vi "DAQConfig.vi"() -> ()   [LabVIEW 2017, in "DAQConfig.lvlib"]
uses:
  DAQConfig.lvlib
  Communication/SubVIs/QueueRepo.Action.ctl
  Main/GUIReferences.Action.ctl
  <vilib>/Utility/miscctls.llb/LVPointTypeDef.ctl
  Communication/Communication.lvlib
  Main/MainGUI.lvlib
panel:
  in  "Start Button":bool
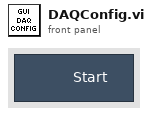
[diagram p1: front panel]
types:
  T1 = typedef "Communication.lvlib/QueueRepo.Action.ctl" = enum16{"Add", "Get", "Destroy", "Get All", "Clear"}
  T2 = typedef "LVPointTypeDef.ctl" = cluster{"Horizontal":i16, "Vertical":i16}
  T3 = typedef "MainGUI.lvlib/GUIReferences.Action.ctl" = enum16{"Get", "Register", "Unregister"}
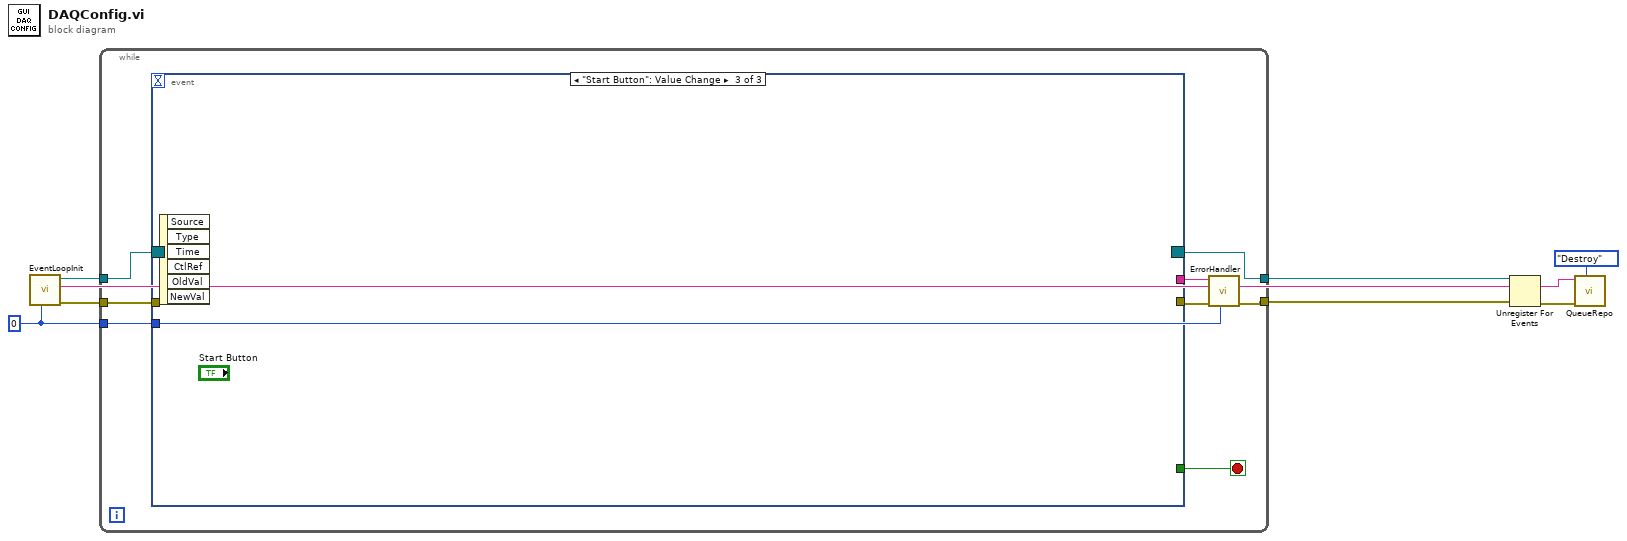
[diagram p0: block diagram]
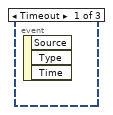
[diagram p2: hidden frame]
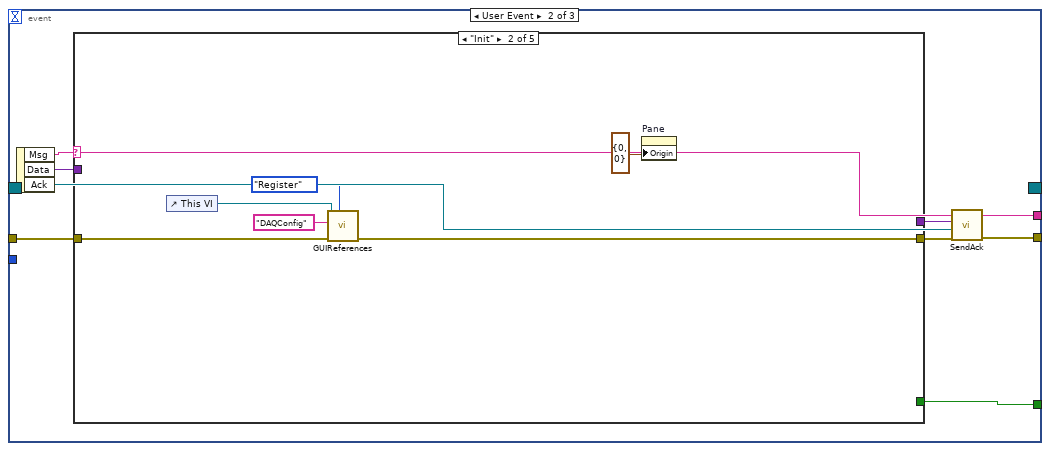
[diagram p3: hidden frame]
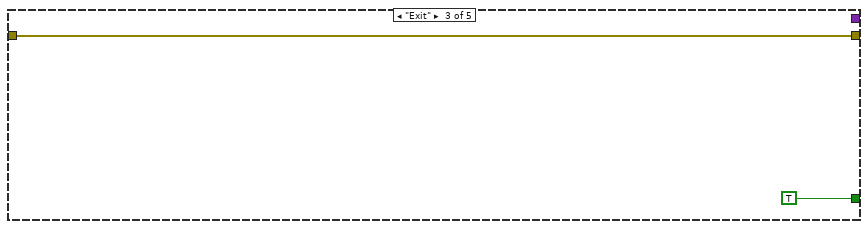
[diagram p5: hidden frame]
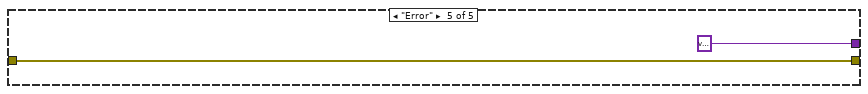
[diagram p7: hidden frame]
diagram:
  w6 = 0 ("Instance")
  n1 = call "EventLoopInit.vi"("Instance"=w6) -> ("error out"=w7:errorcluster, "Loop Name"=w3:string, "Event Registration Refnum"=w8:refnum<event-registration>)  [unwired: 8 in]
  n2 = while {
    tunnel: w8 -> [w16]
    tunnel: w7 -> [w15]
    tunnel: w6 -> [w10]
    tunnel: [w13] -> w5
    tunnel: [w12] -> w4
    stop <- w14 stop-if-true
    n3 = event shown="[2] \"Start Button\": Value Change" {
      selector: w16 -> [_ _ _]
      dyn-events: [_ _ _] -> w13
      timeout: _ -> [_ _ _]
      tunnel: w15 -> [_ w23 _]
      tunnel: [_ w17 _] -> w11
      tunnel: w10 -> [_ _ _]
      tunnel: [_ w19 _] -> w14
      tunnel: [_ w18 _] -> w9
      event Timeout {
        n4 = event-data() -> ()  [unwired: 1 in, 3 out]
      }
      event User Event {
        n5 = event-data() -> ("Msg"=w18:string, "Data"=w24:variant, "Ack"=w22:refnum<notifier>)  [unwired: 1 in]
        n6 = case shown="\"Init\"" w18 {
          tunnel: w24 -> [_ _ _ _ _]
          tunnel: w23 -> [w25 w31 w33 w34 w35]
          tunnel: [_ _ _ _ variant] -> w21
          tunnel: [w25 w30 w33 w34 w35] -> w20
          tunnel: [_ _ TRUE _ _] -> w19
          frame Default {
          }
          frame "Init" {
            n7 = control-ref of="This VI"() -> (w28:refnum<vi>)
            n8 = call "GUIReferences.vi"("Action"=GUIReferences.Action."Register", "error in (no error)"=w31, "String"="DAQConfig", "VI Refnum"=w28) -> ("error out"=w30:errorcluster)  [unwired: 6 in, 1 out]
            n9 = property on="Pane" class="Pane"("Origin"=T2 {"Horizontal"=0, "Vertical"=0}) -> ()  [unwired: 2 in, 2 out]
          }
          frame "Exit" {
          }
          frame "Tick" {
          }
          frame "Error" {
          }
        }
        n10 = call "SendAck.vi"("error in (no error)"=w20, "Ack"=w22, "Variant"=w21) -> ("error out"=w17:errorcluster)  [unwired: 8 in]
      }
      event "Start Button": Value Change {
        n11 = event-data() -> ()  [unwired: 1 in, 6 out]
      }
    }
    n12 = call "ErrorHandler.vi"("Instance"=w10, "error in (no error)"=w11, "Msg"=w9) -> ("error out"=w12:errorcluster)  [unwired: 8 in]
  }
  n13 = Unregister For Events(event registration refnum=w5, error in=w4) -> (error out=w2:errorcluster)
  n14 = call "QueueRepo.vi"("Action"=QueueRepo.Action."Destroy", "error in (no error)"=w2, "Name"=w3) -> ()  [unwired: 5 in, 4 out]
